vi "Animated_dice.vi"() -> ()   [LabVIEW 2019]
panel:
  in  "Stop":bool
  out "Ring 2":u16(ring)
  in  "Roll":bool
  # "ANIMATED DICE APPLICATION"
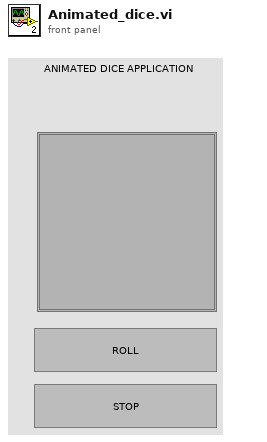
[diagram p1: front panel]
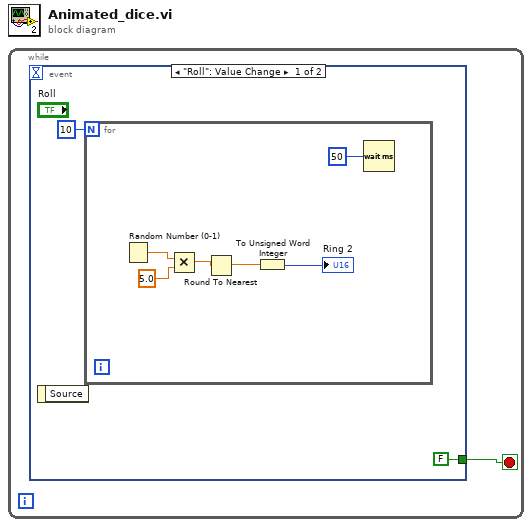
[diagram p0: block diagram]
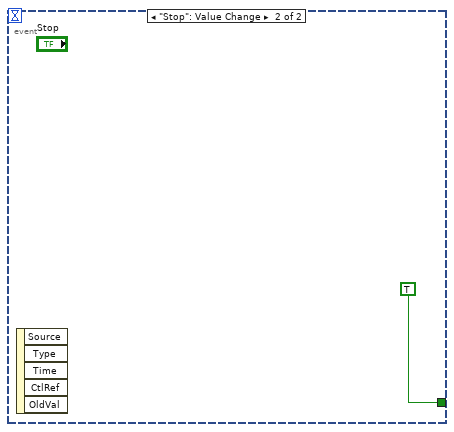
[diagram p2: hidden frame]
diagram:
  n1 = while {
    stop <- w1 stop-if-true
    n2 = event shown="[0] \"Roll\": Value Change" {
      selector: _ -> [_ _]
      dyn-events: _ -> [_ _]
      timeout: _ -> [_ _]
      tunnel: [FALSE TRUE] -> w1
      event "Roll": Value Change {
        n3 = event-data() -> ()  [unwired: 1 in, 1 out]
        n4 = for {
          N: 10 -> [_]
          n5 = Random Number (0-1)() -> (number: 0 to 1=w9:dbl)
          n6 = Multiply(x=w9, y=5.0 ("x")) -> (x*y=w7:dbl)
          n7 = Round To Nearest(number=w7) -> (nearest integer value=w6:dbl)
          n8 = To Unsigned Word Integer(number=w6) -> (unsigned 16bit integer=→"Ring 2":u16)
          n9 = Wait (ms)(milliseconds to wait=u32 50 ("millisecond timer value")) -> ()  [unwired: 1 out]
        }
      }
      event "Stop": Value Change {
        n10 = event-data() -> ()  [unwired: 1 in, 5 out]
      }
    }
  }
